vi "GetAnalyzerParameterValue.vi"(8 "error in":errorcluster, 10 "Parameter Name":string, 11 "connection ID in":refnum<k5>) -> (0 "error out":errorcluster, 1 "Error Info":T1, 2 "Parameter":cluster{"Name":string, "Value":string}, 3 "connection ID out":refnum<k5>, 4 "Log String":string, 5 "OK":bool)   [LabVIEW 2015, in "ProdigyRemoteControl.lvlib"]
uses:
  ProdigyRemoteControl.lvlib
  DEFINITIONS/DEF_RcError.ctl
  DEFINITIONS/DEF_RcCmd.ctl
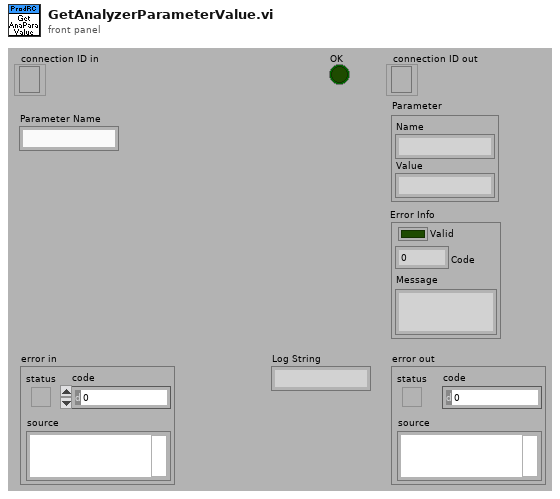
[diagram p1: front panel]
types:
  T1 = typedef "ProdigyRemoteControl.lvlib/DEF_RcError.ctl" = cluster{"Valid":bool, "Code":u16, "Message":string}
  T2 = typedef "ProdigyRemoteControl.lvlib/DEF_RcCmd.ctl" = string
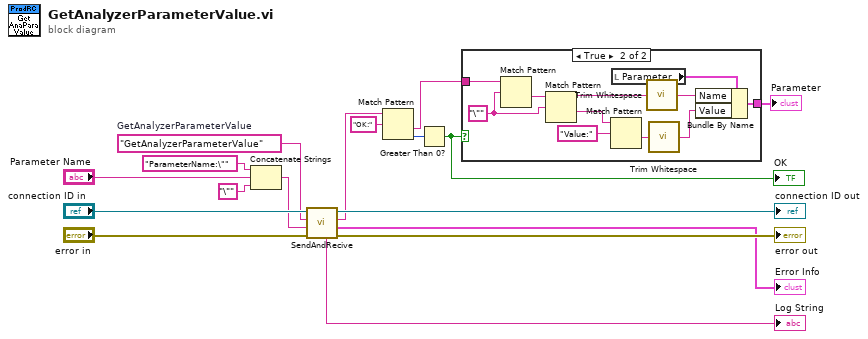
[diagram p0: block diagram]
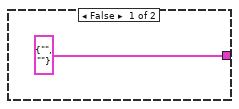
[diagram p2: hidden frame]
diagram:
  w13 = T2 "GetAnalyzerParameterValue"  # GetAnalyzerParameterValue
  n1 = Concatenate Strings("ParameterName:\"" ("string"), "Parameter Name", "\"" ("string")) -> (w7:string)
  n2 = call "SendAndRecive.vi"("error in"="error in", "Parameters"=w7, "Command"=w13, "connection ID in"="connection ID in") -> ("error out"=→"error out":errorcluster, "Error Info"=→"Error Info":T1, "Answer"=w5:string, "connection ID out"=→"connection ID out":refnum<k5>, "Log String"=→"Log String":string)  [unwired: 3 in]
  n3 = Match Pattern(string=w5, regular expression="OK:") -> (after substring=w2:string, offset past match=w4:i32)  [unwired: 1 in, 2 out]
  n4 = Greater Than 0?(x=w4) -> (x > 0?=w1:bool)
  "OK" <- w1
  n5 = case shown="True" w1 {
    tunnel: [cluster{"Name":string, "Value":string} {"Name"="", "Value"=""} ("Parameter") w20] -> w3
    tunnel: w2 -> [_ w19]
    frame False {
    }
    frame True {
      w26 = "\"" ("regular expression")
      n6 = Match Pattern(string=w19, regular expression=w26) -> (after substring=w27:string)  [unwired: 1 in, 3 out]
      n7 = Match Pattern(string=w27, regular expression=w26) -> (before substring=w24:string, after substring=w25:string)  [unwired: 1 in, 2 out]
      n8 = Match Pattern(string=w25, regular expression="Value:") -> (after substring=w28:string)  [unwired: 1 in, 3 out]
      n9 = local read "Parameter"() -> (w23:cluster{"Name":string, "Value":string})
      n10 = call <vilib>:"Trim Whitespace.vi"("string"=w24) -> ("trimmed string"=w22:string)  [unwired: 1 in]
      n11 = call <vilib>:"Trim Whitespace.vi"("string"=w28) -> ("trimmed string"=w21:string)  [unwired: 1 in]
      n12 = Bundle By Name(cluster=w23, "Name"=w22, "Value"=w21) -> (w20:cluster{"Name":string, "Value":string})
    }
  }
  "Parameter" <- w3
